vi "Camera Optics Diagnostics Result_RC.vi"(8 "error in (no error)":errorcluster, 10 "Camera Optics Diagnostics Result":T1={"LightCameraName"="", "DiagnosedImage"=refnum, "DustPercentage"=0.0, "Result"=TRUE}, 11 "Rack Controller in":refnum<class "Rack Controller.lvclass">) -> (0 "error out":errorcluster, 3 "Rack Controller out":refnum<class "Rack Controller.lvclass">)   [LabVIEW 2019, in "Rack Controller.lvclass"]
uses:
  Rack Controller.lvclass
  <vilib>/vision/Image Controls.llb/IMAQ Image.ctl
  Common/Controls/Camera Optics Diagnostics Result.ctl
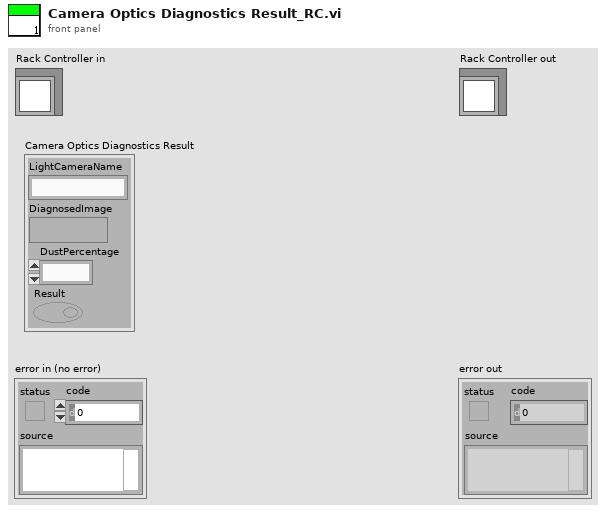
[diagram p1: front panel]
types:
  T1 = typedef "Camera Optics Diagnostics Result.ctl" = cluster{"LightCameraName":string, "DiagnosedImage":T2, "DustPercentage":dbl, "Result":bool}
  T2 = typedef "IMAQ Image.ctl" = refnum<image>
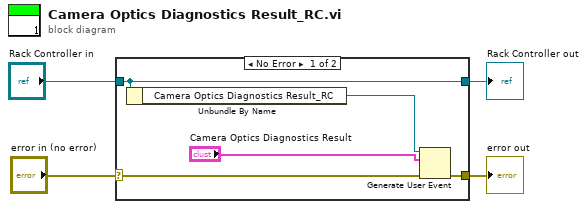
[diagram p0: block diagram]
diagram:
  n1 = case shown="No Error" "error in (no error)" {
    selector: "error in (no error)" -> [w6 w11]
    tunnel: [w5 w11] -> w3
    tunnel: [w9 w10] -> w1
    tunnel: "Rack Controller in" -> [w9 w10]
    frame No Error {
      n2 = Unbundle By Name(w9) -> ("Camera Optics Diagnostics Result_RC"=w8:refnum<user-event>)
      n3 = Generate User Event(user event=w8, event data cluster="Camera Optics Diagnostics Result", error in=w6) -> (error out=w5:errorcluster)  [unwired: 1 in, 1 out]
    }
    frame Error {
    }
  }
  "error out" <- w3
  "Rack Controller out" <- w1
